vi "4 -2 - Extarct non repeated combined transition data rally seperated.vi"() -> ()   [LabVIEW 2013]
uses:
  <vilib>/Utility/file.llb/Read From Spreadsheet File (string).vi
panel:
  out "Bottom player":string[](array[string])
  in  "Rally seperated transition data":path
  out "Top player":string[](array[string])
  out "both players non repeated transitions":string[][](array[string])
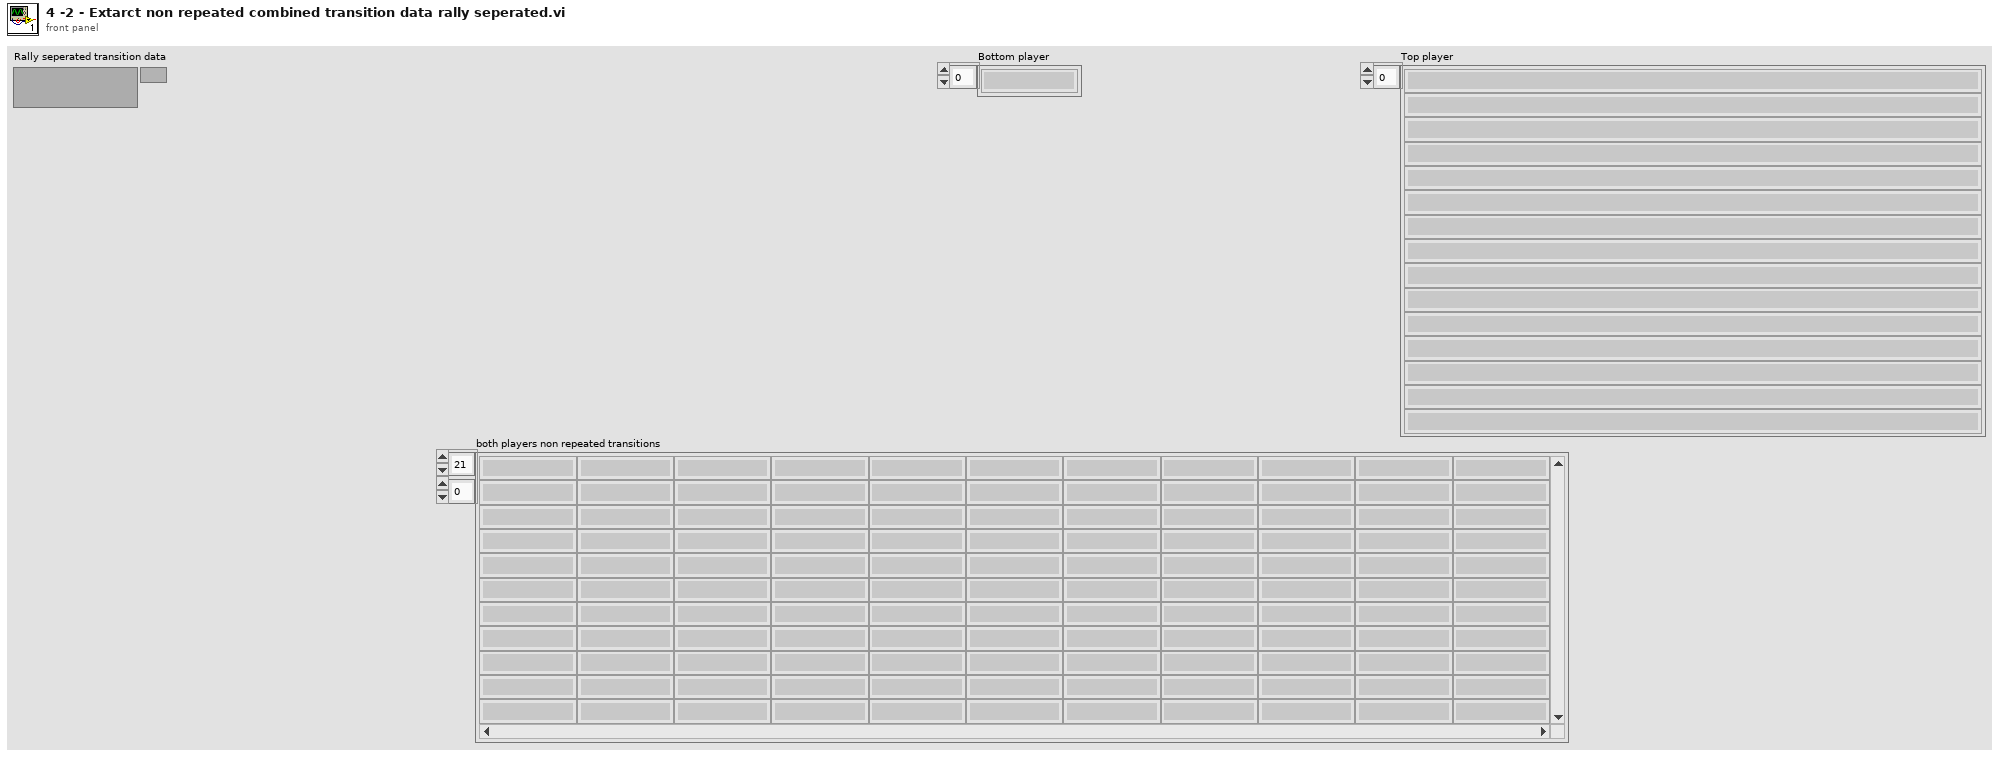
[diagram p1: front panel]
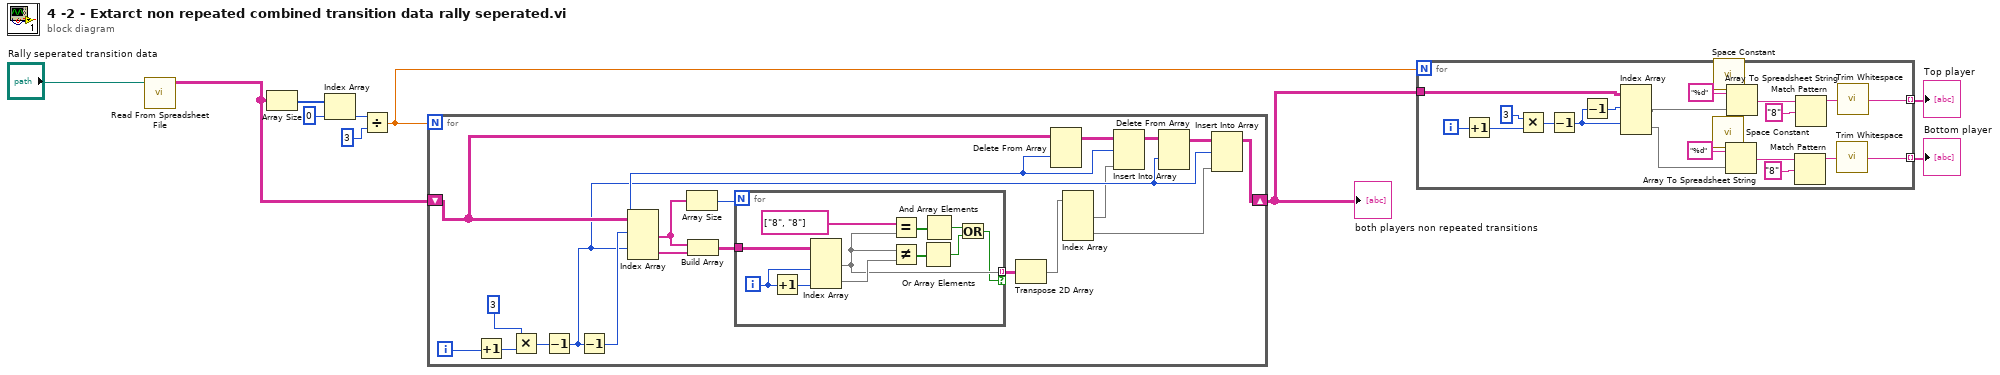
[diagram p0: block diagram]
diagram:
  n1 = call-poly <vilib>:"Read From Spreadsheet File.vi"("file path (dialog if empty)"="Rally seperated transition data") -> ("all rows"=w2:string[][])  [unwired: 6 in, 4 out]
  n2 = Array Size(array=w2) -> (size(s)=w10:i32[])
  n3 = Index Array(array=w10, index=0) -> (element=w8:i32)
  n4 = Divide(x=w8, y=3) -> (x/y=w6:dbl)
  n5 = for {
    N: w6 -> [_]
    shift-right: [w12] -> w5
    shift-left: w2 -> [w19]
    i -> [w29]
    n6 = Increment(x=w29) -> (x+1=w28:i32)
    n7 = Multiply(x=3, y=w28) -> (x*y=w26:i32)
    n8 = Decrement(x=w26) -> (x-1=w13:i32)
    n9 = Decrement(x=w13) -> (x-1=w17:i32)
    n10 = Index Array(array=w19, index (row) #1=w17, index (row) #2=w13) -> (element #1=w23:string[], element #2=w25:string[])  [unwired: 2 in]
    n11 = Array Size(array=w23) -> (size(s)=w22:i32)
    n12 = Build Array(w23, w25) -> (w24:string[][])
    n13 = for {
      N: w22 -> [_]
      tunnel: w24 -> [w40]
      tunnel: [w35] -> w21 mode=indexing if=w30
      i -> [w37]
      n14 = Increment(x=w37) -> (x+1=w39:i32)
      n15 = Index Array(array=w40, index (col) #1=w37, index (col) #2=w39) -> (element #1=w35:string[], element #2=w38:string[])  [unwired: 2 in]
      n16 = Equal?(x=string[] ["8", "8"], y=w35) -> (x = y?=w32:bool[])
      n17 = Not Equal?(x=w35, y=w38) -> (x != y?=w36:bool[])
      n18 = Or Array Elements(Boolean array=w36) -> (logical OR=w33:bool)
      n19 = And Array Elements(Boolean array=w32) -> (logical AND=w31:bool)
      n20 = Or(x=w31, y=w33) -> (x .or. y?=w30:bool)
    }
    n21 = Transpose 2D Array(2D array=w21) -> (transposed array=w20:string[][])
    n22 = Delete From Array(array=w19, index (row)=w17) -> (array with subset deleted=w18:string[][])  [unwired: 2 in, 1 out]
    n23 = Index Array(array=w20) -> (element #1=w11:string[], element #2=w14:string[])  [unwired: 4 in]
    n24 = Insert Into Array(array=w18, index (row)=w17, new element=w11) -> (w16:string[][])  [unwired: 1 in]
    n25 = Delete From Array(array=w16, index (row)=w13) -> (array with subset deleted=w15:string[][])  [unwired: 2 in, 1 out]
    n26 = Insert Into Array(array=w15, index (row)=w13, new element=w14) -> (w12:string[][])  [unwired: 1 in]
  }
  "both players non repeated transitions" <- w5
  n27 = for {
    N: w6 -> [_]
    tunnel: w5 -> [w55]
    tunnel: [w50] -> w4 mode=indexing
    tunnel: [w41] -> w1 mode=indexing
    i -> [w58]
    n28 = Increment(x=w58) -> (x+1=w59:i32)
    n29 = Multiply(x=3, y=w59) -> (x*y=w61:i32)
    n30 = Decrement(x=w61) -> (x-1=w56:i32)
    n31 = Decrement(x=w56) -> (x-1=w57:i32)
    n32 = Index Array(array=w55, index (row) #1=w57, index (row) #2=w56) -> (element #1=w48:string[], element #2=w42:string[])  [unwired: 2 in]
    n33 = call <vilib>:"Space Constant.vi"() -> ("String"=w47:string)
    n34 = call <vilib>:"Space Constant.vi"() -> ("String"=w49:string)
    n35 = Array To Spreadsheet String(delimiter (Tab)=w47, array=w42, 3:"%d" ("format string")) -> (spreadsheet string=w45:string)
    n36 = Array To Spreadsheet String(delimiter (Tab)=w49, array=w48, 3:"%d" ("format string")) -> (spreadsheet string=w52:string)
    n37 = Match Pattern(string=w45, regular expression="8") -> (before substring=w43:string)  [unwired: 1 in, 3 out]
    n38 = Match Pattern(string=w52, regular expression="8") -> (before substring=w54:string)  [unwired: 1 in, 3 out]
    n39 = call <vilib>:"Trim Whitespace.vi"("string"=w43) -> ("trimmed string"=w41:string)  [unwired: 1 in]
    n40 = call <vilib>:"Trim Whitespace.vi"("string"=w54) -> ("trimmed string"=w50:string)  [unwired: 1 in]
  }
  "Top player" <- w4
  "Bottom player" <- w1
